vi "Start.vi"(8 "error in (no error)":errorcluster, 11 "TimeStamper in":refnum<class "TimeStamper.lvclass">) -> (0 "error out":errorcluster, 3 "TimeStamper out":refnum<class "TimeStamper.lvclass">)   [LabVIEW 2010, in "TimeStamper.lvclass"]
uses:
  TimeStamper.lvclass
  TimeStamper.lvclass/TimeStamper.ctl
  <vilib>/DAQmx/write.llb/DAQmx Write (Digital Bool 1Line 1Point).vi
  <vilib>/DAQmx/create/channels.llb/DAQmx Create Channel (DO-Digital Output).vi
  <vilib>/daqmx/miscellaneous.llb/DAQmx Fill In Error Info.vi
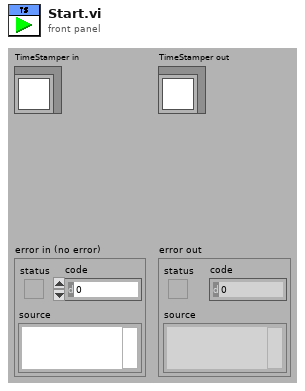
[diagram p1: front panel]
types:
  T1 = cluster{"Read Access":enum8{"Allowed", "Required", "None"}, "Write Access":enum8{"Allowed", "Required", "None"}}
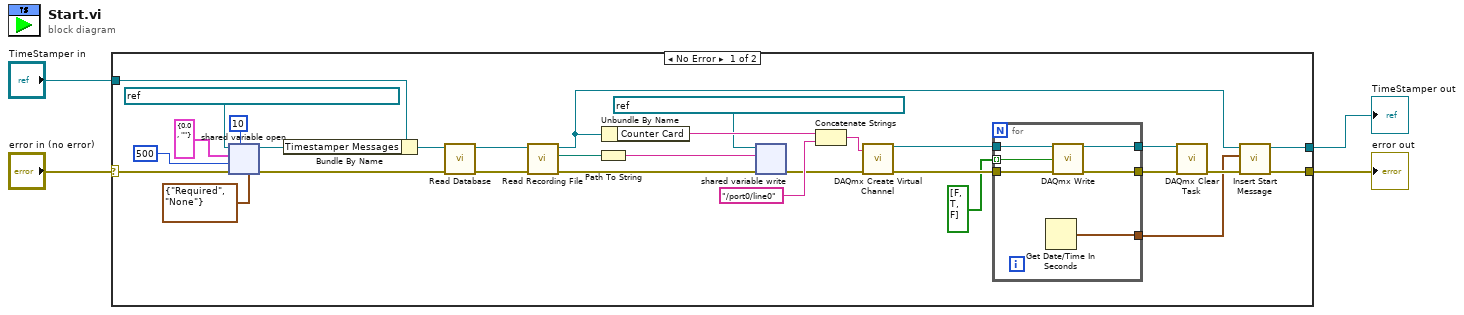
[diagram p0: block diagram]
diagram:
  n1 = case shown="No Error" "error in (no error)" {
    selector: "error in (no error)" -> [w16 w42]
    tunnel: [w11 w42] -> w3
    tunnel: [w13 w41] -> w1
    tunnel: "TimeStamper in" -> [w17 w41]
    frame No Error {
      n2 = shared-variable-open(refnum<k21> "ni.var.psp://localhost/AcquisitionVariables/Message" ("shared variable refnum in"), w16, cluster{"Channel":dbl, "Message":string} {"Channel"=0.0, "Message"=""} ("Message"), T1 {"Read Access"=enum."Required", "Write Access"=enum."None"} ("access"), 500 ("timeout ms"), u32 10 ("buffer size in elements")) -> (w23:refnum<k21>, w15:errorcluster)
      n3 = Bundle By Name(cluster=w17, "Timestamper Messages"=w23) -> (w14:refnum<class "TimeStamper.lvclass">)
      n4 = call-dynamic "Read Database.vi"("error in (no error)"=w15, "AcquistionObject in"=w14) -> ("error out"=w5:errorcluster, "AcquistionObject out"=w9:refnum<class "TimeStamper.lvclass">)  [unwired: 7 in, 1 out]
      n5 = call-dynamic "Read Recording File.vi"("error in (no error)"=w5, "AcquistionObject in"=w9) -> ("error out"=w6:errorcluster, "Recording File"=w7:path, "AcquistionObject out"=w8:refnum<class "TimeStamper.lvclass">)  [unwired: 7 in]
      n6 = Path To String(path=w7) -> (string=w20:string)
      n7 = Unbundle By Name(w8) -> ("Counter Card"=w34:tag)
      n8 = shared-variable-write(refnum<k21> "ni.var.psp://localhost/AcquisitionVariables/SessionPath" ("shared variable refnum in"), w6, w20) -> (w19:errorcluster)  [unwired: 1 out]
      n9 = Concatenate Strings(w34, "/port0/line0" ("string")) -> (w32:string)
      n10 = call-poly <vilib>:"DAQmx Create Virtual Channel.vi"("lines"=w32, "error in"=w19) -> ("task out"=w29:refnum<k21>, "error out"=w31:errorcluster)  [unwired: 12 in]
      n11 = for {
        tunnel: w31 -> [w40]
        tunnel: [w39] -> w30
        tunnel: w29 -> [w38]
        tunnel: [w37] -> w28
        tunnel: bool[] [FALSE, TRUE, FALSE] -> [w36] mode=indexing
        tunnel: [w35] -> w10
        n12 = Get Date/Time In Seconds() -> (seconds since 1Jan1904=w35:timestamp)
        n13 = call-poly <vilib>:"DAQmx Write.vi"("task/channels in"=w38, "data"=w36, "error in"=w40) -> ("task out"=w37:refnum<k21>, "error out"=w39:errorcluster)  [unwired: 10 in, 1 out]
      }
      n14 = call <vilib>:"DAQmx Clear Task.vi"("task in"=w28, "error in"=w30) -> ("error out"=w12:errorcluster)  [unwired: 13 in]
      n15 = call-dynamic "Insert Start Message.vi"("error in (no error)"=w12, "Start Time"=w10, "TimeStamper in"=w8) -> ("error out"=w11:errorcluster, "TimeStamper out"=w13:refnum<class "TimeStamper.lvclass">)  [unwired: 7 in]
    }
    frame Error {
    }
  }
  "error out" <- w3
  "TimeStamper out" <- w1
